vi "list selected files.vi"(1 "Ring":u16(ring) items=["#.xml_decay of spotxxx.dat", "#_decay of spotxxx.dat"], 2 "selection path":path) -> (0 "path names":path[](array[path]))   [LabVIEW 2009]
uses:
  <vilib>/Utility/file.llb/Read From Spreadsheet File (DBL).vi
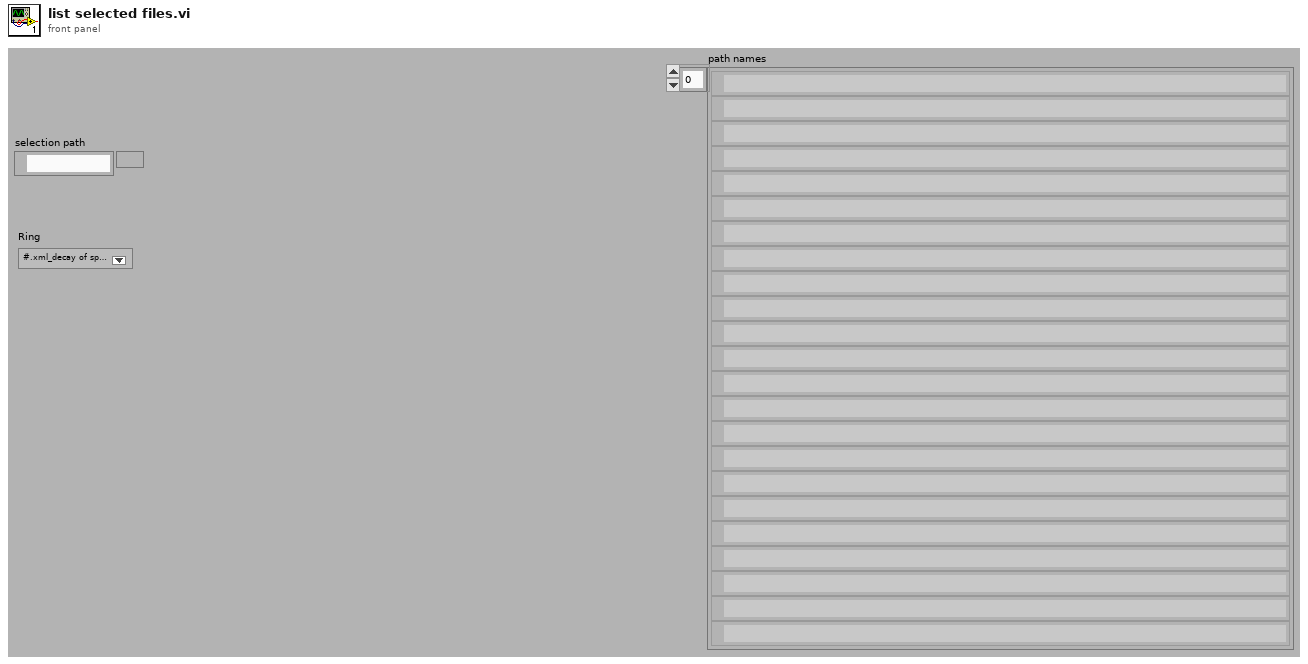
[diagram p1: front panel]
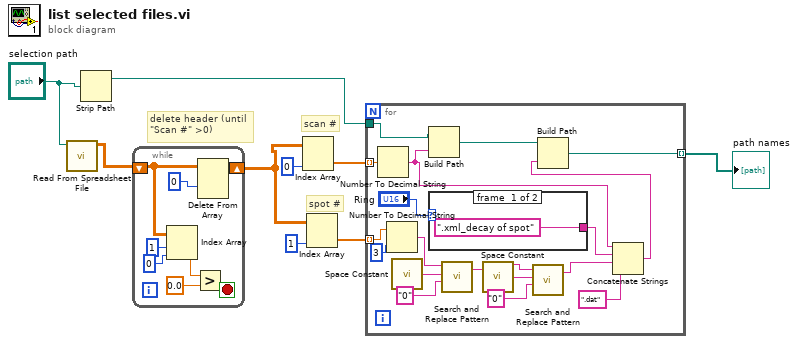
[diagram p0: block diagram]
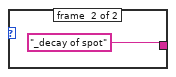
[diagram p2: hidden frame]
diagram:
  # "delete header (until\n\"Scan #\" >0)"
  # "spot #"
  # "scan #"
  n1 = call-poly <vilib>:"Read From Spreadsheet File.vi"("file path (dialog if empty)"="selection path") -> ("all rows"=w3:dbl[][])  [unwired: 6 in, 4 out]
  n2 = Strip Path(path="selection path") -> (stripped path=w4:path)  [unwired: 1 out]
  n3 = while {
    shift-right: [w17] -> w2
    shift-left: w3 -> [w15]
    stop <- w11 stop-if-true
    n4 = Index Array(array=w15, index (row)=1 ("disabled index (row)"), index (col)=0 ("disabled index (col)")) -> (element=w12:dbl)
    n5 = Greater?(x=w12, y=0.0) -> (0:w11:bool)
    n6 = Delete From Array(array=w15, index (row)=0) -> (array with subset deleted=w17:dbl[][])  [unwired: 2 in, 1 out]
  }
  n7 = Index Array(array=w2, index (col)=0 ("disabled index (col)")) -> (element=w7:dbl[])  [unwired: 1 in]
  n8 = Index Array(array=w2, index (col)=1 ("disabled index (col)")) -> (element=w6:dbl[])  [unwired: 1 in]
  n9 = for {
    tunnel: w7 -> [w35] mode=indexing
    tunnel: w6 -> [w34] mode=indexing
    tunnel: w4 -> [w24]
    tunnel: [w20] -> w1 mode=indexing
    n10 = Number To Decimal String(number=w35) -> (decimal integer string=w23:string)  [unwired: 1 in]
    n11 = Number To Decimal String(number=w34, width (-)=i16 3) -> (decimal integer string=w32:string)
    n12 = call <vilib>:"Space Constant.vi"() -> ("String"=w31:string)
    n13 = Build Path(base path=w24, name or relative path=w23) -> (appended path=w22:path)
    n14 = case shown="1" "Ring" {
      tunnel: [".xml_decay of spot" "_decay of spot"] -> w18
      frame #0 {
      }
      frame #1 {
      }
    }
    n15 = call <vilib>:"Search and Replace Pattern.vi"("string"=w32, "regular expression (\"\")"=w31, "replace string (\"\")"="0") -> ("result string"=w26:string)  [unwired: 2 in, 1 out]
    n16 = call <vilib>:"Space Constant.vi"() -> ("String"=w28:string)
    n17 = call <vilib>:"Search and Replace Pattern.vi"("string"=w26, "regular expression (\"\")"=w28, "replace string (\"\")"="0") -> ("result string"=w25:string)  [unwired: 2 in, 1 out]
    n18 = Concatenate Strings(w23, w18, w25, ".dat" ("string")) -> (w21:string)
    n19 = Build Path(base path=w22, name or relative path=w21) -> (appended path=w20:path)
  }
  "path names" <- w1
